vi "GYRO_TEST.vi"() -> ()   [LabVIEW 2010]
uses:
  subVIs/dIMU_Gyro_dps.vi
panel:
  in  "stop":bool
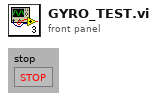
[diagram p1: front panel]
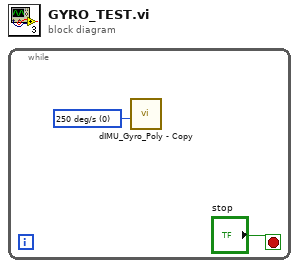
[diagram p0: block diagram]
diagram:
  n1 = while {
    stop <- "stop" stop-if-true
    w2 = u8 0 items=["250 deg/s"=0, "500 deg/s"=16, "2000 deg/s"=32] ("Gyro Scale")
    n2 = call-poly "dIMU_Gyro_Poly - Copy.vi"("Gyro Scale"=w2) -> ()  [unwired: 7 in, 4 out]
  }
